vi "Manual - Invert (SubVI).vi"(8 "error in (no error)":errorcluster, 11 "Cluster":T1 {"PID"."Output Range"."Low" format="%.2f"; "PID"."Output Range"."High" format="%.2f"; "PID"."PID Tuning"."(Td, min)" format="%.6f"; "PID"."PID Tuning"."(Ti, min)" format="%.6f"; "PID"."PID Tuning"."(Kc)" format="%.6f"}) -> (0 "error out":errorcluster, 1 "Run":bool, 2 "Machine":i32, 3 "Speed":u32, 5 "Dir":bool)   [LabVIEW 2019]
uses:
  Controls/Manual - Data Structure.ctl
  Controls/FGV States.ctl
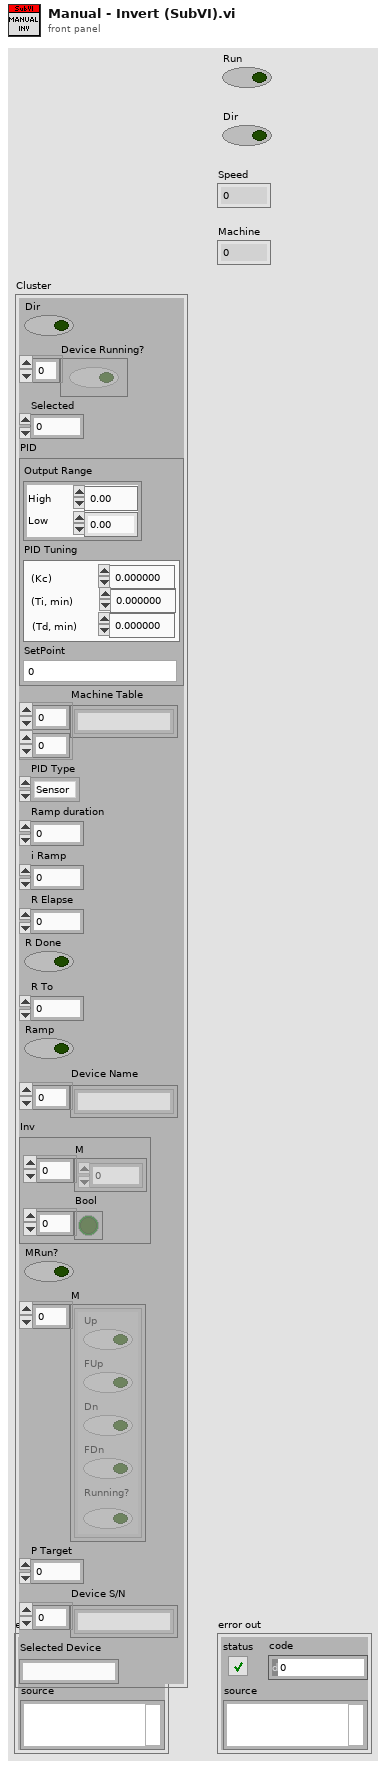
[diagram p1: front panel]
types:
  T1 = typedef "Manual - Data Structure.ctl" = cluster{"Dir":bool, "Device Running?":bool[], "Selected":u16, "PID":cluster{"Output Range":cluster{"High":dbl, "Low":dbl}, "PID Tuning":cluster{"(Kc)":dbl, " (Ti, min)":dbl, "(Td, min)":dbl}, "SetPoint":dbl}, "Machine Table":string[][], "PID Type":enum32{"Sensor", "Displacement"}, "Ramp duration":i32, "i Ramp":i32, "R Elapse":dbl, "R Done":bool, "R To":dbl, "Ramp":bool, "Device Name":string[], "Inv":cluster{"M":i32[], "Bool":bool[]}, "MRun?":bool, "M":cluster{"Up":bool, "FUp":bool, "Dn":bool, "FDn":bool, "Running?":bool}[], "P Target":dbl, "Device S/N":string[], "Selected Device":string}
  T2 = typedef "FGV States.ctl" = enum16{"Read", "Write"}
  T3 = cluster{"Up":bool, "FUp":bool, "Dn":bool, "FDn":bool, "Running?":bool}[]
  T4 = cluster{"Up":bool, "FUp":bool, "Dn":bool, "FDn":bool, "Running?":bool}
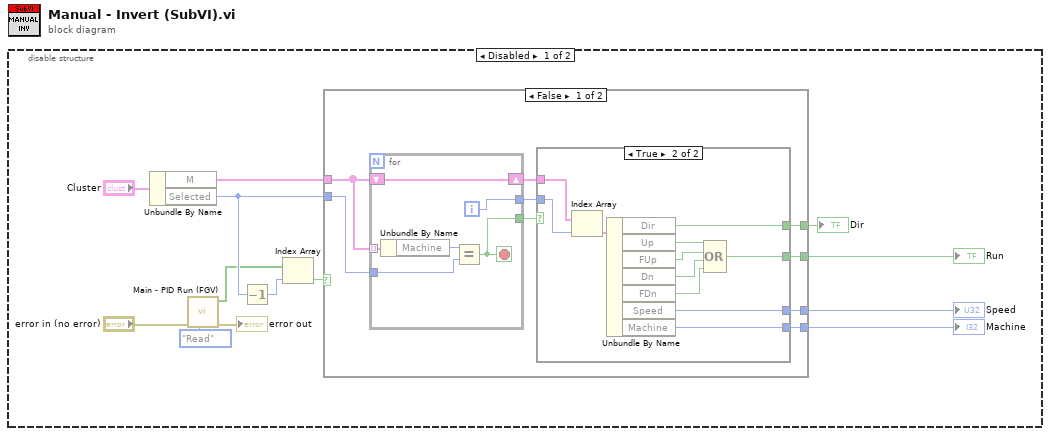
[diagram p0: block diagram]
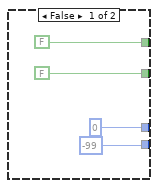
[diagram p2: hidden frame]
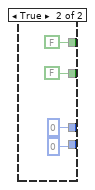
[diagram p3: hidden frame]
diagram:
  n1 = disable-structure shown="Disabled" {
    frame Disabled {
      n2 = Unbundle By Name("Cluster") -> ("M"=w1:T3, "Selected"=w6:u16)
      n3 = call "Main - PID Run (FGV).vi"("Action"=FGV_States."Read", "error In"="error in (no error)") -> ("error out"=→"error out":errorcluster, "Button ref out"=w4:bool[])  [unwired: 8 in]
      n4 = Decrement(x=w6) -> (x-1=w5:u16)
      n5 = Index Array(array=w4, index=w5) -> (element=w7:bool)
      n6 = case shown="False" w7 {
        tunnel: w1 -> [w22 _]
        tunnel: w6 -> [w19 _]
        tunnel: [w17 FALSE] -> w10
        tunnel: [w16 u32 0 ("Speed")] -> w8
        tunnel: [w15 0 ("Machine")] -> w9
        tunnel: [w14 FALSE ("Dir")] -> w13
        frame False {
          n7 = for {
            tunnel: w22 -> [w43] mode=indexing
            tunnel: w19 -> [w41]
            tunnel: [w40] -> w21
            shift-right: [w39] -> w20
            shift-left: w22 -> [w39]
            tunnel: [w38] -> w18
            i -> [w40]
            stop <- w38 stop-if-true
            n8 = Unbundle By Name(w43) -> ("Machine"=w42:i32)
            n9 = Equal?(x=w42, y=w41) -> (x = y?=w38:bool)
          }
          n10 = case shown="True" w18 {
            tunnel: w21 -> [_ w36]
            tunnel: w20 -> [_ w37]
            tunnel: [FALSE w32] -> w17
            tunnel: [FALSE ("Dir") w27] -> w14
            tunnel: [u32 0 ("Speed") w31] -> w16
            tunnel: [-99 ("Machine") w30] -> w15
            frame False {
            }
            frame True {
              n11 = Index Array(array=w37, index=w36) -> (element=w35:T4)
              n12 = Unbundle By Name(w35) -> ("Dir"=w27:bool, "Up"=w34:bool, "FUp"=w33:bool, "Dn"=w29:bool, "FDn"=w28:bool, "Speed"=w31:u32, "Machine"=w30:i32)
              n13 = Compound Arithmetic op=OR(w34, w33, w29, w28) -> (w32:bool)
            }
          }
        }
        frame True {
        }
      }
      "Dir" <- w13
      "Run" <- w10
      "Machine" <- w9
      "Speed" <- w8
    }
    frame Enabled {
    }
  }
